vi "Control_Panel_Execute.vi"() -> ()   [LabVIEW 2019]
uses:
  Globals/Control_Panel_Globals.vi
panel:
  in  "time_to_run":u32
  in  "Spinwheel_Throttle":dbl
  out "Spin_Wheel_Motor":dbl
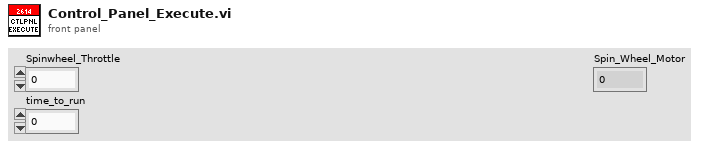
[diagram p1: front panel]
types:
  T1 = typedef "Control_Panel_Cluster.ctl" = cluster{"Control_State":enum16{"No-Op", "Rotational_Control", "Positional_Control", "Manual_Control"}, "Start_Movement":bool, "Abort":bool, "Rotation_Control?":bool, "Positional_Control? ":bool, "Throttle":dbl}
  T2 = enum16{"No-Op", "Rotational_Control", "Positional_Control", "Manual_Control"}
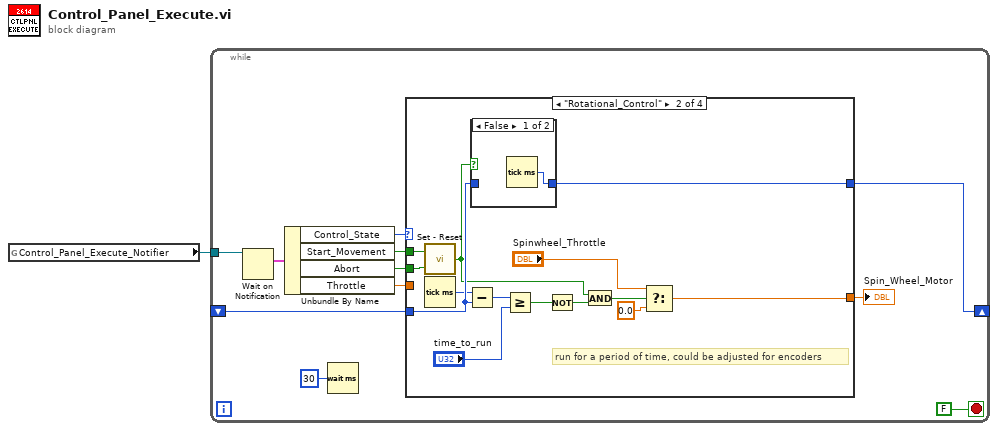
[diagram p0: block diagram]
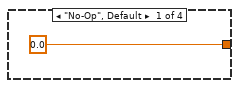
[diagram p2: hidden frame]
diagram:
  n1 = global read "Control_Panel_Globals.vi" "Control_Panel_Execute_Notifier"() -> (w1:refnum<notifier>)
  n2 = while {
    tunnel: w1 -> [w12]
    shift-right: [w5] -> _
    shift-left: _ -> [w4]
    stop <- FALSE stop-if-true
    n3 = Wait on Notification(notifier=w12) -> (notification=w11:T1)  [unwired: 3 in, 3 out]
    n4 = Unbundle By Name(w11) -> ("Control_State"=w10:T2, "Start_Movement"=w7:bool, "Abort"=w6:bool, "Throttle"=w8:dbl)
    n5 = Wait (ms)(milliseconds to wait=u32 30) -> ()  [unwired: 1 out]
    n6 = case shown="\"Rotational_Control\"" w10 {
      tunnel: [0.0 ("Spin_Wheel_Speed") w14 _ w30] -> w9
      tunnel: w8 -> [_ _ _ w30]
      tunnel: w7 -> [_ w27 _ _]
      tunnel: w6 -> [_ w26 _ _]
      tunnel: [_ w24 _ _] -> w5
      tunnel: w4 -> [_ w21 _ _]
      frame "No-Op", Default {
      }
      frame "Rotational_Control" {
        # "run for a period of time, could be adjusted for encoders"
        n7 = call "Set - Reset.vi"("Reset"=w26, "Set"=w27) -> ("Output"=w19:bool)
        n8 = Tick Count (ms)() -> (millisecond timer value=w20:u32)
        n9 = Subtract(x=w20, y=w21) -> (x-y=w23:u32)
        n10 = case shown="False" w19 {
          tunnel: [w28 w29] -> w24
          tunnel: w21 -> [_ w29]
          frame False {
            n11 = Tick Count (ms)() -> (millisecond timer value=w28:u32)
          }
          frame True {
          }
        }
        n12 = Greater Or Equal?(x=w23, y="time_to_run") -> (x >= y?=w18:bool)
        n13 = Not(x=w18) -> (.not. x?=w17:bool)
        n14 = And(x=w19, y=w17) -> (x .and. y?=w16:bool)
        n15 = Select(t="Spinwheel_Throttle", s=w16, f=0.0) -> (s? t:f=w14:dbl)
      }
      frame "Positional_Control" {
        # "SPINNING LOGIC, color offsets"
      }
      frame "Manual_Control" {
      }
    }
    "Spin_Wheel_Motor" <- w9
  }
